vi "Open File.vi"(7 "Operation":T1, 8 "error in (no error)":errorcluster, 11 "Path":path) -> (0 "error out":errorcluster, 3 "ConfigFile out":refnum<class "ConfigFile.lvclass">)   [LabVIEW 2017, in "ImportExport.lvlib"]
uses:
  ImportExport.lvlib
  ConfigFile/ConfigFile.lvclass
  Operation.ctl
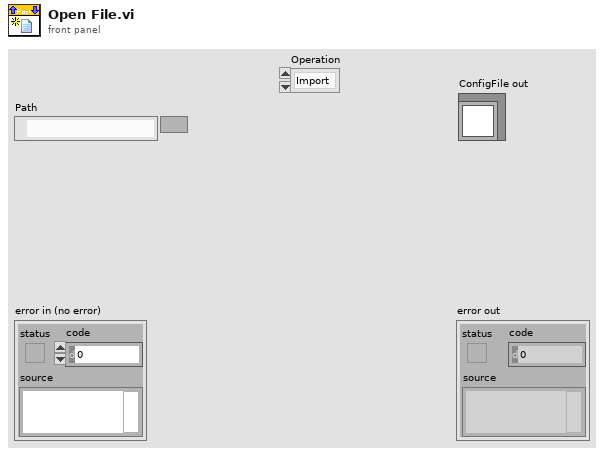
[diagram p1: front panel]
types:
  T1 = typedef "ImportExport.lvlib/Operation.ctl" = enum16{"Import", "Export"}
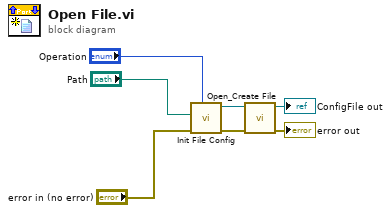
[diagram p0: block diagram]
diagram:
  n1 = call "Init File Config.vi"("Operation"="Operation", "error in (no error)"="error in (no error)", "Path"="Path") -> ("error out"=w5:errorcluster, "ConfigFile out"=w7:refnum<class "ConfigFile.lvclass">)  [unwired: 7 in]
  n2 = call-dynamic "Open_Create File.vi"("error in (no error)"=w5, "ConfigFile in"=w7) -> ("error out"=→"error out":errorcluster, "ConfigFile out"=→"ConfigFile out":refnum<class "ConfigFile.lvclass">)  [unwired: 6 in, 2 out]
